vi "encodeCluster.vi"(8 "error in (no error)":errorcluster, 10 "Variant":variant) -> (0 "error out":errorcluster, 2 "Array":u8[](array[numeric]) format="%.0x")   [LabVIEW 2016, in "MsgPack.lvlib"]
uses:
  MsgPack.lvlib
  <vilib>/Utility/error.llb/Error Cluster From Error Code.vi
  <vilib>/ErrorRing/Error Ring.xnode
  <vilib>/Utility/Data Type/NI_Data Type.lvlib
panel:
  out "Element Names":string[](array[string])
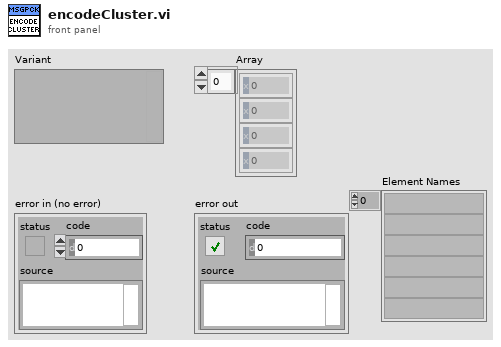
[diagram p1: front panel]
types:
  T1 = typedef "NI_Data Type.lvlib/Data Type.ctl" = enum8{"Invalid Type", "Void", "I8", "I16", "I32", "I64", "U8", "U16", "U32", "U64", "Single Float", "Double Float", "Extended Float", "Single Complex", "Double Complex", "Extended Complex", "Enum U8", "Enum U16", "Enum U32", "Enum U64", "Single Float With Unit", "Double Float With Unit", "Extended Float With Unit", "Single Complex with Unit", "Double Complex with Unit", "Extended Complex with Unit", "Boolean", "String", "Path", "Picture", "Tag", "Array", "Cluster", "Variant", "LV Variant", "Waveform", "Timestamp", "Digital Waveform", "Digital Data", "ExpressData", "Refnum", "External Data", "VI", "Poly VI", "LabVIEW Class Instance", "Fixed Point"}
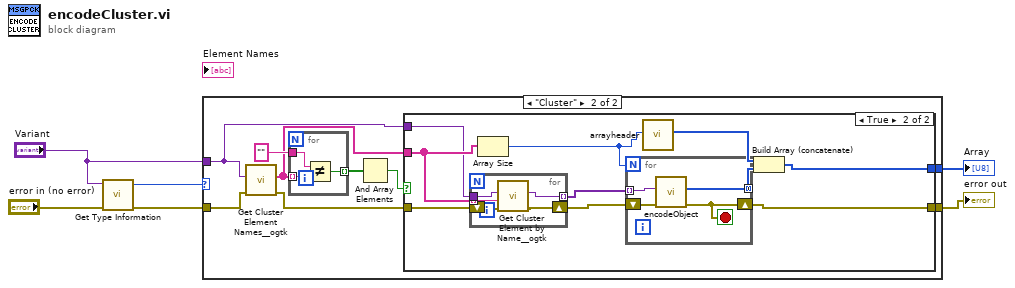
[diagram p0: block diagram]
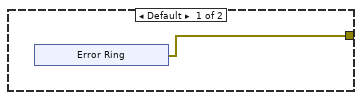
[diagram p2: hidden frame]
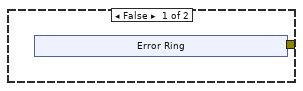
[diagram p3: hidden frame]
diagram:
  n1 = call <vilib>:"Get Type Information.vi"("error in (no error)"="error in (no error)", "Variant"="Variant") -> ("error out"=w4:errorcluster, "Type"=w5:T1)  [unwired: 5 in, 3 out]
  n2 = case shown="\"Cluster\"" w5 {
    tunnel: w4 -> [_ w19]
    tunnel: "Variant" -> [_ w14]
    tunnel: [_ w21] -> w3
    tunnel: [w7 w20] -> w2
    frame Default {
      n3 = xnode "Error Ring"() -> ("error out"=w7:errorcluster)
    }
    frame "Cluster" {
      n4 = call <userlib>:"Get Cluster Element Names__ogtk.vi"("error in (no error)"=w19, "Cluster"=w14) -> ("error out"=w18:errorcluster, "Element Names"=w13:string[])  [unwired: 8 in]
      n5 = for {
        tunnel: w13 -> [w49] mode=indexing
        tunnel: "" ("x") -> [w48]
        tunnel: [w47] -> w16 mode=indexing
        n6 = Not Equal?(x=w48, y=w49) -> (x != y?=w47:bool)
      }
      n7 = And Array Elements(Boolean array=w16) -> (logical AND=w15:bool)
      n8 = case shown="True" w15 {
        tunnel: [_ w35] -> w21
        tunnel: [w22 w34] -> w20
        tunnel: w18 -> [_ w33]
        tunnel: w14 -> [_ w31]
        tunnel: w13 -> [_ w32]
        frame False {
          n9 = xnode "Error Ring"() -> ("error out"=w22:errorcluster)
        }
        frame True {
          n10 = for {
            tunnel: w32 -> [w41] mode=indexing
            shift-right: [w39] -> w30
            shift-left: w33 -> [w42]
            tunnel: w31 -> [w40]
            tunnel: [w38] -> w29 mode=indexing
            n11 = call <userlib>:"Get Cluster Element by Name__ogtk.vi"("error in (no error)"=w42, "Element Name"=w41, "Cluster"=w40) -> ("error out"=w39:errorcluster, "VElement"=w38:variant)  [unwired: 6 in, 1 out]
          }
          n12 = Array Size(array=w32) -> (size(s)=w28:i32)
          n13 = for {
            N: w28 -> [_]
            tunnel: w29 -> [w46] mode=indexing
            shift-right: [w43] -> w34
            shift-left: w30 -> [w45]
            tunnel: [w44] -> w36 mode=concatenating
            stop <- w43 stop-if-true
            n14 = call "encodeObject.vi"("error in (no error)"=w45, "Variant"=w46) -> ("error out"=w43:errorcluster, "Array"=w44:u8[])  [unwired: 8 in]
          }
          n15 = call "arrayheader.vi"("Numeric"=w28) -> ("header"=w37:u8[])  [unwired: 10 in]
          n16 = Build Array (concatenate)(w37, w36) -> (w35:u8[])
        }
      }
    }
  }
  "Array" <- w3
  "error out" <- w2
